vi "Read barcode prototype.vi"() -> ()   [LabVIEW 2013]
uses:
  Controls/ALTS-2015 Scanner Driver Options.ctl
panel:
  in  "Scanner 2?  (Scanner1)":bool
  out "Serial No":string
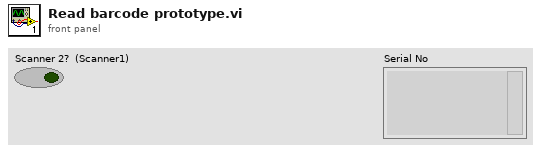
[diagram p1: front panel]
types:
  T1 = typedef "ALTS-2015 Scanner Driver Options.ctl" = enum16{"Initialize Scanner", "Read Scanner", "Close Scanner"}
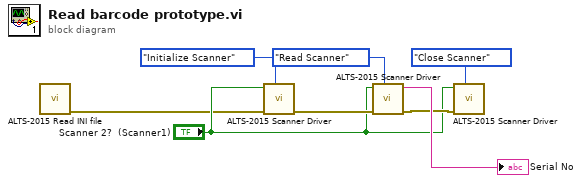
[diagram p0: block diagram]
diagram:
  n1 = call "ALTS-2015 Read INI file.vi"() -> ("error out"=w1:errorcluster)  [unwired: 11 in]
  n2 = call "ALTS-2015 Scanner Driver.vi"("Operation"=ALTS-2015_Scanner_Driver_Options."Initialize Scanner", "error in (no error)"=w1, "Scanner 2?  (Scanner1)"="Scanner 2?  (Scanner1)") -> ("error out"=w3:errorcluster)  [unwired: 7 in, 1 out]
  n3 = call "ALTS-2015 Scanner Driver.vi"("Operation"=ALTS-2015_Scanner_Driver_Options."Read Scanner", "error in (no error)"=w3, "Scanner 2?  (Scanner1)"="Scanner 2?  (Scanner1)") -> ("error out"=w4:errorcluster, "Serial No"=→"Serial No":string)  [unwired: 7 in]
  n4 = call "ALTS-2015 Scanner Driver.vi"("Operation"=ALTS-2015_Scanner_Driver_Options."Close Scanner", "error in (no error)"=w4, "Scanner 2?  (Scanner1)"="Scanner 2?  (Scanner1)") -> ()  [unwired: 7 in, 2 out]
